vi "dfd_FLP Lattice Normalized Section.vi"(2 "^k(m)":dbl format="%.2f", 3 "k(m)":dbl format="%.2f", 4 "w(m-1)":dbl format="%.2f", 5 "x(m)":dbl format="%.2f") -> (0 "w(m)":dbl format="%.2f", 1 "x(m-1)":dbl format="%.2f")   [LabVIEW 2017, in "NI_DigFilter_FXP.lvlib"]
uses:
  <vilib>/addons/Digital Filter Design/NI_DigFilter_FXP.lvlib
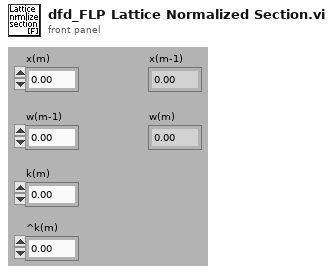
[diagram p1: front panel]
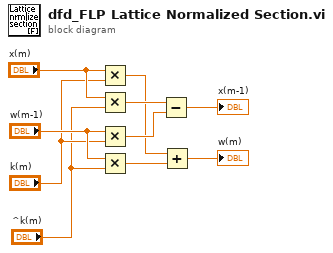
[diagram p0: block diagram]
diagram:
  n1 = Multiply(x="x(m)", y="k(m)") -> (x*y=w2:dbl)
  n2 = Multiply(x="x(m)", y="^k(m)") -> (x*y=w6:dbl)
  n3 = Multiply(x="w(m-1)", y="k(m)") -> (x*y=w5:dbl)
  n4 = Multiply(x="w(m-1)", y="^k(m)") -> (x*y=w3:dbl)
  n5 = Subtract(x=w6, y=w5) -> (x-y=→"x(m-1)":dbl)
  n6 = Add(x=w2, y=w3) -> (x+y=→"w(m)":dbl)
